vi "Master Program.vi"() -> ()   [LabVIEW 2018]
uses:
  <vilib>/Instr/_visa.llb/VISA Configure Serial Port (Instr).vi
  Instance           3 22Saved   Master Program .vi
  Instance          12 22Saved   Master Program .vi
  Instance          11 22Saved   Master Program .vi
  <vilib>/express/express shared/transition.llb/Dynamic To Waveform Array.vi
  <vilib>/express/express arith-compare/Formula/Block/exnFormulaBlock how many pts in the wave.vi
  <vilib>/express/express shared/ex_Modify Signal Name.vi
  <vilib>/express/express shared/transition.llb/Waveform Array To Dynamic.vi
  Instance          10 22Saved   Master Program .vi
  Instance           8 22Saved   Master Program .vi
  Instance           6 22Saved   Master Program .vi
  Instance           4 22Saved   Master Program .vi
  <vilib>/express/express arith-compare/Formula/XNode/ExpressFormulaBlockNode.xnode
panel:
  out "Room Temperature":dbl
  out "Temperature 85 C":dbl
  out "Temperature 40 C":dbl
  out "Wheatstone":dbl
  out "Voltage 2":dbl
  out "Voltage 1":dbl
  in  "STOP":bool
  out "16:1 SWITCH  #":i32
  out "8:1 MUX SWITCH #":i32
  in  "Arduino Serial Port":refnum<visa-resource-name>="VXI0::0::INSTR"
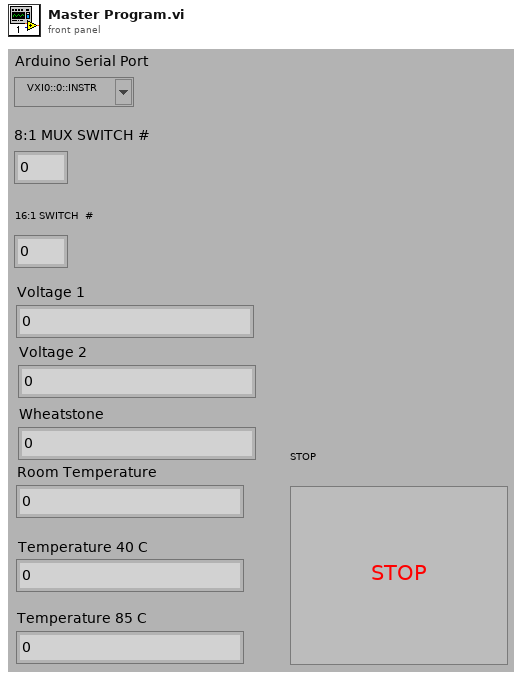
[diagram p1: front panel]
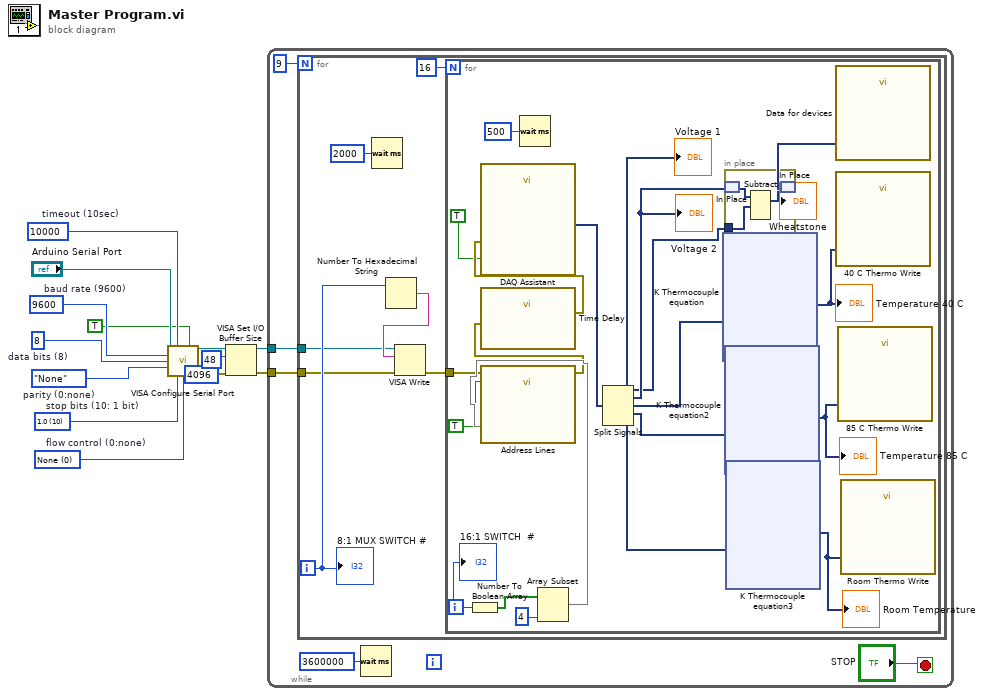
[diagram p0: block diagram]
diagram:
  w14 = u16 8  # data bits (8)
  w12 = u16 0 items=["None"=0, "XON/XOFF"=1, "RTS/CTS"=2, "DTR/DSR"=4, "XON/XOFF & RTS/CTS"=3, "XON/XOFF & DTR/DSR"=5]  # flow control (0:none)
  w11 = u16 10 items=["1.0"=10, "1.5"=15, "2.0"=20]  # stop bits (10: 1 bit)
  w10 = u32 10000  # timeout (10sec)
  w9 = enum16{"None", "Odd", "Even", "Mark", "Space"}."None"  # parity (0:none)
  w8 = u32 9600  # baud rate (9600)
  n1 = call-poly "VISA Configure Serial Port"("VISA resource name"="Arduino Serial Port", "timeout (10sec)"=w10, "Enable Termination\nChar (T)"=TRUE ("Enable Termination\nChar (T)"), "baud rate (9600)"=w8, "data bits (8)"=w14, "parity (0:none)"=w9, "stop bits (10: 1 bit)"=w11, "flow control (0:none)"=w12) -> ("VISA resource name out"=w5:refnum<visa-resource-name>, "error out"=w6:errorcluster)  [unwired: 6 in]
  n2 = VISA Set I/O Buffer Size(VISA resource name=w5, mask (16)=u16 48, size (4096)=u32 4096, error in (no error)=w6) -> (VISA resource name out=w3:refnum<visa-resource-name>, error out=w4:errorcluster)
  n3 = while {
    tunnel: w3 -> [w16]
    tunnel: w4 -> [w15]
    stop <- "STOP" stop-if-true
    n4 = for {
      N: 9 -> [_]
      tunnel: w16 -> [w21]
      tunnel: w15 -> [w20]
      i -> [w25]
      n5 = Wait (ms)(milliseconds to wait=u32 2000) -> ()  [unwired: 1 out]
      n6 = Number To Hexadecimal String(2:w25) -> (0:w26:string)  [unwired: 1 in]
      n7 = VISA Write(VISA resource name=w21, write buffer=w26, error in (no error)=w20) -> (error out=w23:errorcluster)  [unwired: 2 out]
      n8 = for {
        N: 16 -> [_]
        tunnel: w23 -> [w29]
        i -> [w43]
        n9 = Number To Boolean Array(number=w43) -> (Boolean array=w45:bool[])
        n10 = Wait (ms)(milliseconds to wait=u32 500) -> ()  [unwired: 1 out]
        n11 = Array Subset(array=w45, length=4) -> (w44:bool[])  [unwired: 1 in]
        n12 = call "Address Lines"("stop (T)"=TRUE, "data"=w44, "error in"=w29) -> ("error out"=w38:errorcluster)  [unwired: 7 in, 1 out]
        n13 = call "Time Delay"("error in (no error)"=w38) -> ("error out"=w37:errorcluster)  [unwired: 10 in]
        n14 = call "DAQ Assistant"("stop (F)"=TRUE, "error in"=w37) -> ("data"=w40:dynamicdata)  [unwired: 7 in, 2 out]
        n15 = Split Signals(w40) -> (w41:dynamicdata, w42:dynamicdata, w33:dynamicdata, w32:dynamicdata, w31:dynamicdata)  [unwired: 5 in]
        "Voltage 1" <- w41
        "Voltage 2" <- w42
        n16 = xnode "K Thermocouple equation"("V"=w33) -> ("결과"=w34:dynamicdata)  [unwired: 1 in, 1 out]
        "Temperature 40 C" <- w34
        n17 = in-place {
          in-place-border: w41 -> [w465]
          n18 = in-place-match #1(w42) -> (w466:dynamicdata)
          n19 = Subtract(1:w465, 2:w466) -> (0:w464:dynamicdata)  [unwired: 1 in, 1 out]
          n20 = in-place-match #1(w464) -> (w27:dynamicdata)
        }
        "Wheatstone" <- w27
        n21 = xnode "K Thermocouple equation2"("V"=w32) -> ("결과"=w35:dynamicdata)  [unwired: 1 in, 1 out]
        "Temperature 85 C" <- w35
        n22 = xnode "K Thermocouple equation3"("V"=w31) -> ("결과"=w36:dynamicdata)  [unwired: 1 in, 1 out]
        "Room Temperature" <- w36
        n23 = call "Data for devices"("Signals"=w27) -> ()  [unwired: 8 in, 3 out]
        n24 = call "40 C Thermo Write"("Signals"=w34) -> ()  [unwired: 8 in, 3 out]
        n25 = call "85 C Thermo Write"("Signals"=w35) -> ()  [unwired: 8 in, 3 out]
        n26 = call "Room Thermo Write"("Signals"=w36) -> ()  [unwired: 8 in, 3 out]
        "16:1 SWITCH  #" <- w43
      }
      "8:1 MUX SWITCH #" <- w25
    }
    n27 = Wait (ms)(milliseconds to wait=u32 3600000) -> ()  [unwired: 1 out]
  }
